vi "Preview Selected Waveform.vi"(8 "error in (no error)":errorcluster, 10 "Waveform Listbox Ref":refnum<vi>, 11 "Data In":T1 {"Toggle Channels"."Initial State" items=["High"=101, "Low"=102]; "Sample Rate" format="%.2p"}) -> (0 "error out":errorcluster, 2 "Selected Waveform":waveform(dbl)(graph), 3 "Data Out":T1 {"Toggle Channels"."Initial State" items=["High"=101, "Low"=102]; "Sample Rate" format="%.2p"})   [LabVIEW 2021]
uses:
  Controls/Data.ctl
  Controls/Script Trigger Routing.ctl
  Controls/Toggle Channel.ctl
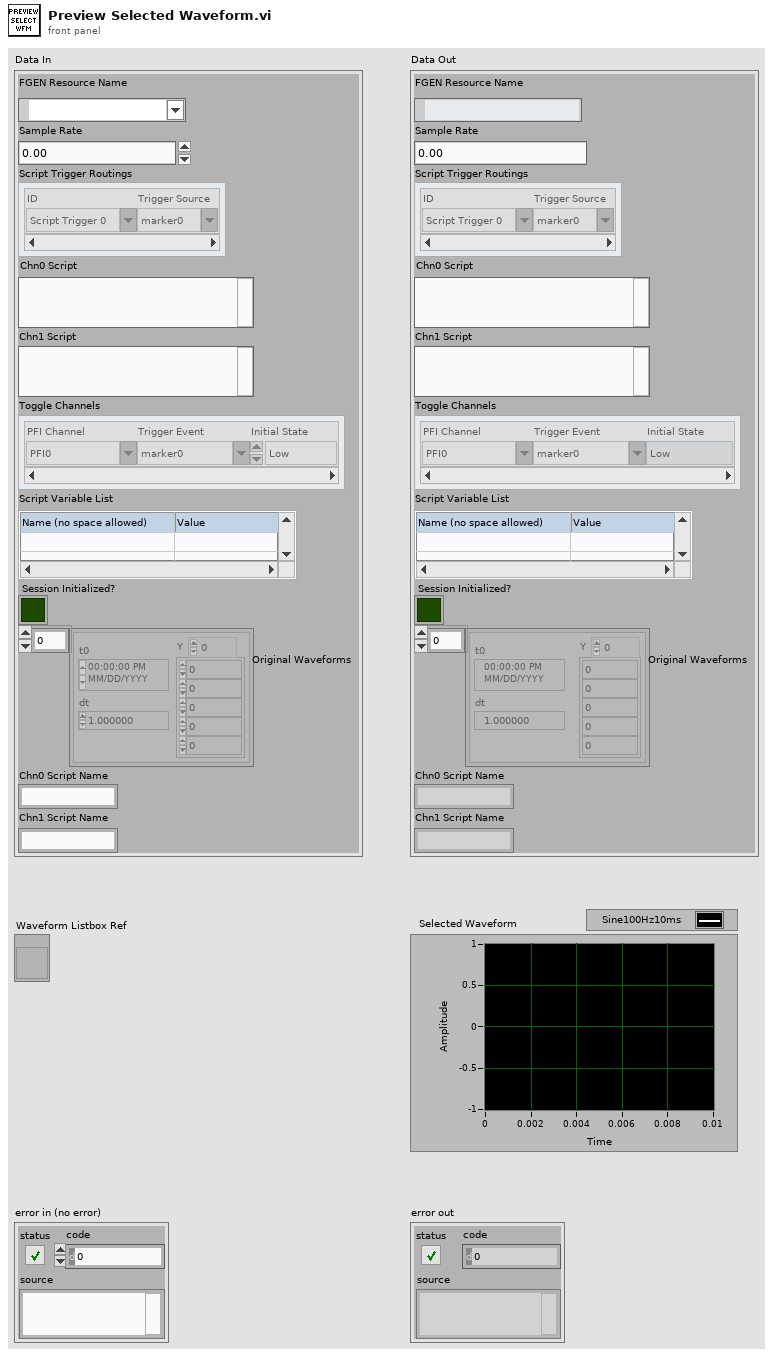
[diagram p1: front panel]
types:
  T1 = typedef "Data.ctl" = cluster{"FGEN Resource Name":refnum<k15>, "Sample Rate":dbl, "Script Trigger Routings":T2[], "Chn0 Script":string, "Chn1 Script":string, "Toggle Channels":T3[], "Script Variable List":string[][], "Session Initialized?":bool, "Original Waveforms":waveform(dbl)[], "Chn0 Script Name":string, "Chn1 Script Name":string}
  T2 = typedef "Script Trigger Routing.ctl" = cluster{"ID":string, "Trigger Source":string}
  T3 = typedef "Toggle Channel.ctl" = cluster{"PFI Channel":string, "Trigger Event":string, "Initial State":u16}
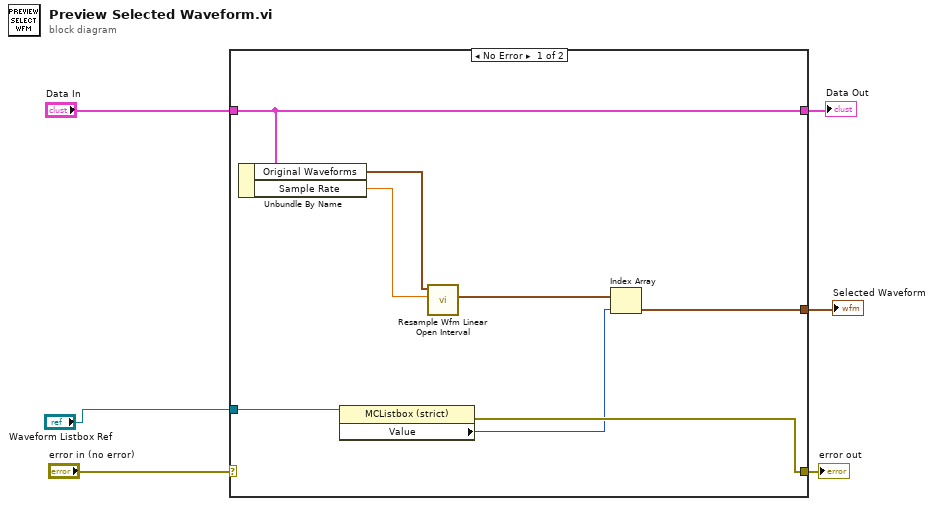
[diagram p0: block diagram]
diagram:
  n1 = case shown="No Error" "error in (no error)" {
    selector: "error in (no error)" -> [_ w16]
    tunnel: "Data In" -> [w14 w15]
    tunnel: [w14 w15] -> w5
    tunnel: [w11 w16] -> w3
    tunnel: "Waveform Listbox Ref" -> [w13 _]
    tunnel: [w12 _] -> w1
    frame No Error {
      n2 = Unbundle By Name(w14) -> ("Original Waveforms"=w9:waveform(dbl)[], "Sample Rate"=w8:dbl)
      n3 = property class="MCListbox (strict)"(reference=w13) -> (error out=w11:errorcluster, "Value"=w10:i32)  [unwired: 1 in, 1 out]
      n4 = call "Resample Wfm Linear Open Interval.vi"("Sample Rate"=w8, "Original Waveforms"=w9) -> ("Resampled Waveform"=w7:waveform(dbl)[])  [unwired: 8 in, 1 out]
      n5 = Index Array(array=w7, index=w10) -> (element=w12:waveform(dbl))
    }
    frame Error {
    }
  }
  "Data Out" <- w5
  "error out" <- w3
  "Selected Waveform" <- w1
